vi "Validate Scope Horizontal Timing.vi"(8 "error in (no error)":errorcluster, 11 "scope info map":T3(c390)) -> (0 "error out":errorcluster)   [LabVIEW 2021, in "PMIC Common.lvlib"]
uses:
  PMIC Common.lvlib
  Scope Parameters.ctl
  <instrlib>/niScope/Controls/niScope vertical coupling.ctl
  <vilib>/ErrorRing/Error Ring.xnode
  <vilib>/Utility/error.llb/Error Cluster From Error Code.vi
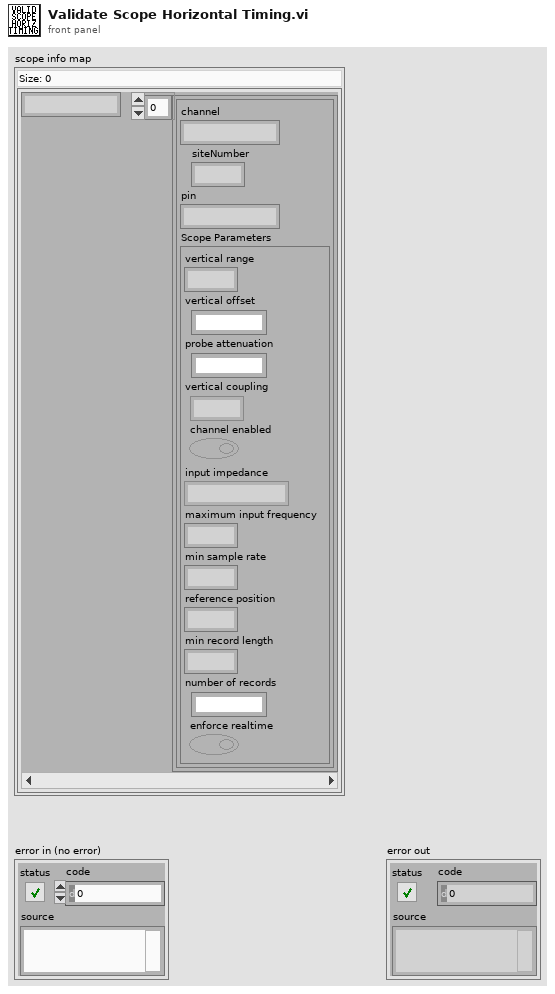
[diagram p1: front panel]
types:
  T1 = typedef "PMIC Common.lvlib/Scope Parameters.ctl" = cluster{"vertical range":dbl, "vertical offset":dbl, "probe attenuation":dbl, "vertical coupling":T2, "channel enabled":bool, "input impedance":u32, "maximum input frequency":dbl, "min sample rate":dbl, "reference position":dbl, "min record length":i32, "number of records":i32, "enforce realtime":bool}
  T2 = typedef "niScope vertical coupling.ctl" = i32
  T3 = map{string, cluster{"channel":string, "siteNumber":i32, "pin":string, "Scope Parameters":T1}[]}
  T4 = cluster{"channel":string, "siteNumber":i32, "pin":string, "Scope Parameters":T1}[]
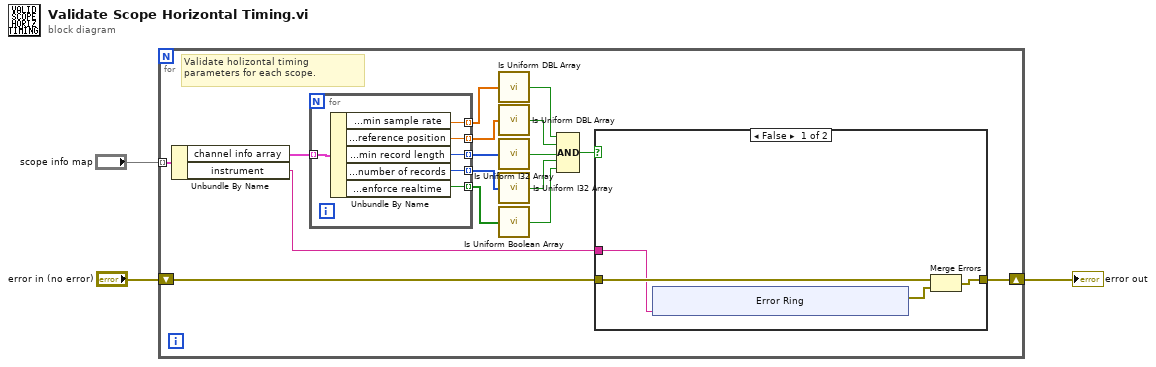
[diagram p0: block diagram]
diagram:
  n1 = for {
    tunnel: "scope info map" -> [w19] mode=indexing
    shift-right: [w5] -> w2
    shift-left: "error in (no error)" -> [w4]
    # "Validate holizontal timing parameters for each scope."
    n2 = Unbundle By Name(w19) -> ("channel info array"=w18:T4, "instrument"=w6:string)
    n3 = for {
      tunnel: w18 -> [w37] mode=indexing
      tunnel: [w36] -> w17 mode=indexing
      tunnel: [w35] -> w16 mode=indexing
      tunnel: [w34] -> w15 mode=indexing
      tunnel: [w33] -> w14 mode=indexing
      tunnel: [w32] -> w13 mode=indexing
      n4 = Unbundle By Name(w37) -> ("Scope Parameters.min sample rate"=w36:dbl, "Scope Parameters.reference position"=w35:dbl, "Scope Parameters.min record length"=w34:i32, "Scope Parameters.number of records"=w33:i32, "Scope Parameters.enforce realtime"=w32:bool)
    }
    n5 = call "Is Uniform DBL Array.vi"("Array"=w17) -> ("Is Uniform Array"=w12:bool)
    n6 = call "Is Uniform DBL Array.vi"("Array"=w16) -> ("Is Uniform Array"=w10:bool)
    n7 = call "Is Uniform I32 Array.vi"("Array"=w15) -> ("Is Uniform Array"=w11:bool)
    n8 = call "Is Uniform I32 Array.vi"("Array"=w14) -> ("Is Uniform Array"=w8:bool)
    n9 = call "Is Uniform Boolean Array.vi"("Array"=w13) -> ("Is Uniform Array"=w9:bool)
    n10 = Compound Arithmetic op=AND(w12, w10, w11, w8, w9) -> (w7:bool)
    n11 = case shown="False" w7 {
      tunnel: w6 -> [w20 _]
      tunnel: [w23 w31] -> w5
      tunnel: w4 -> [w22 w31]
      frame False {
        n12 = xnode "Error Ring"("parameter 0"=w20) -> ("error out"=w21:errorcluster)
        n13 = Merge Errors(w22, w21) -> (w23:errorcluster)
      }
      frame True {
      }
    }
  }
  "error out" <- w2
